vi "TKPS252XG Configure Current-Voltage24.vi"(1 "voltage limit":dbl format="%.2f", 4 "error in (no error)":errorcluster, 5 "current limit":dbl format="%.3f", 6 "channel (ch1:0)":u16(ring) items=["channel 1", "channel 2", "channel 3"], 7 "VISA session":refnum<visa-resource-name>) -> (0 "error out":errorcluster, 3 "dup VISA session":refnum<visa-resource-name>)   [LabVIEW 2024]
doc: "This vi sets the voltage and current settings of the power supply for each of the output channels."
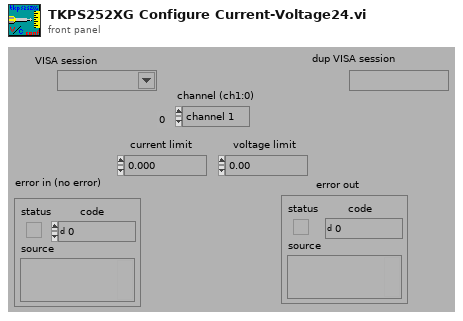
[diagram p1: front panel]
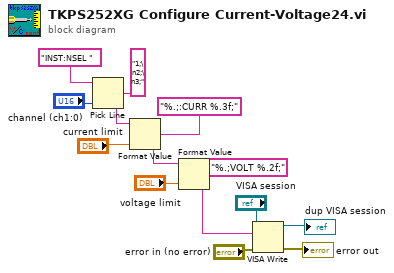
[diagram p0: block diagram]
diagram:
  n1 = Pick Line(string ("")="INST:NSEL " ("VI name"), multi-line string="1;\n2;\n3;" ("VI name"), line index="channel (ch1:0)") -> (output string=w3:string)
  n2 = Format Value(string ("")=w3, format string="%.;:CURR %.3f;", value (0)="current limit") -> (output string=w6:string)
  n3 = Format Value(string ("")=w6, format string="%.;VOLT %.2f;", value (0)="voltage limit") -> (output string=w1:string)
  n4 = VISA Write(VISA resource name="VISA session", write buffer=w1, error in (no error)="error in (no error)") -> (VISA resource name out=→"dup VISA session":refnum<visa-resource-name>, error out=→"error out":errorcluster)  [unwired: 1 out]
